vi "getPastFutureData.vi"(3 "2015 data future - R55 parsed.csv":path, 5 "2015 data past - R55 parsed.csv":path) -> (0 "Data Past Cluster":T1, 2 "Data Future Cluster":T2)   [LabVIEW 2013]
uses:
  <vilib>/Utility/file.llb/Read From Spreadsheet File (DBL).vi
panel:
  # "Daily Past Data       -7               -6              -5              -4              -3               -2              -1"
  # "Daily Future Data +1               +2              +3             +4             +5              +6              +7              +8             +9           +10            +11           +12"
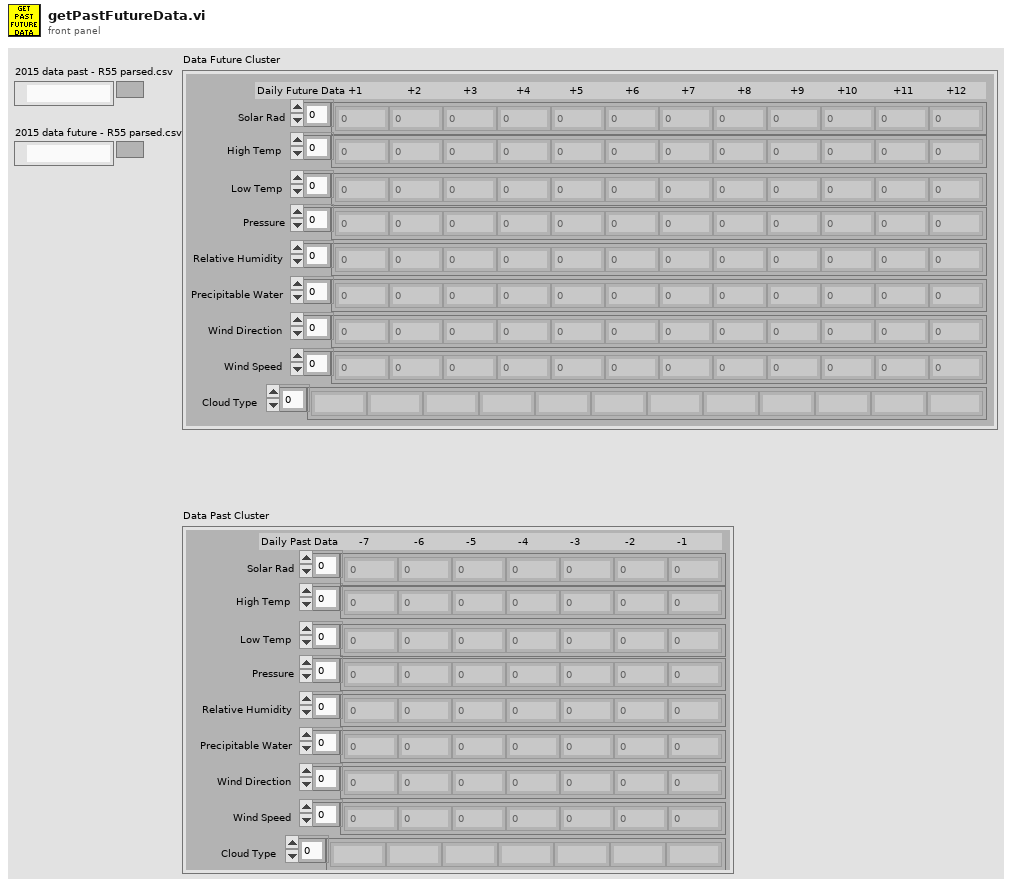
[diagram p1: front panel]
types:
  T1 = cluster{"Wind Speed":dbl[], "Wind Direction":dbl[], "Precipitable Water":dbl[], "Relative Humidity":dbl[], "Pressure":dbl[], "Low Temp":dbl[], "High Temp":dbl[], "Solar Rad":dbl[], "Cloud Type":string[]}
  T2 = cluster{"Solar Rad":dbl[], "High Temp":dbl[], "Low Temp":dbl[], "Pressure":dbl[], "Relative Humidity":dbl[], "Precipitable Water":dbl[], "Wind Direction":dbl[], "Wind Speed":dbl[], "Cloud Type":string[]}
  T3 = cluster{dbl[], dbl[], dbl[], dbl[], dbl[], dbl[], dbl[], dbl[], string[]}
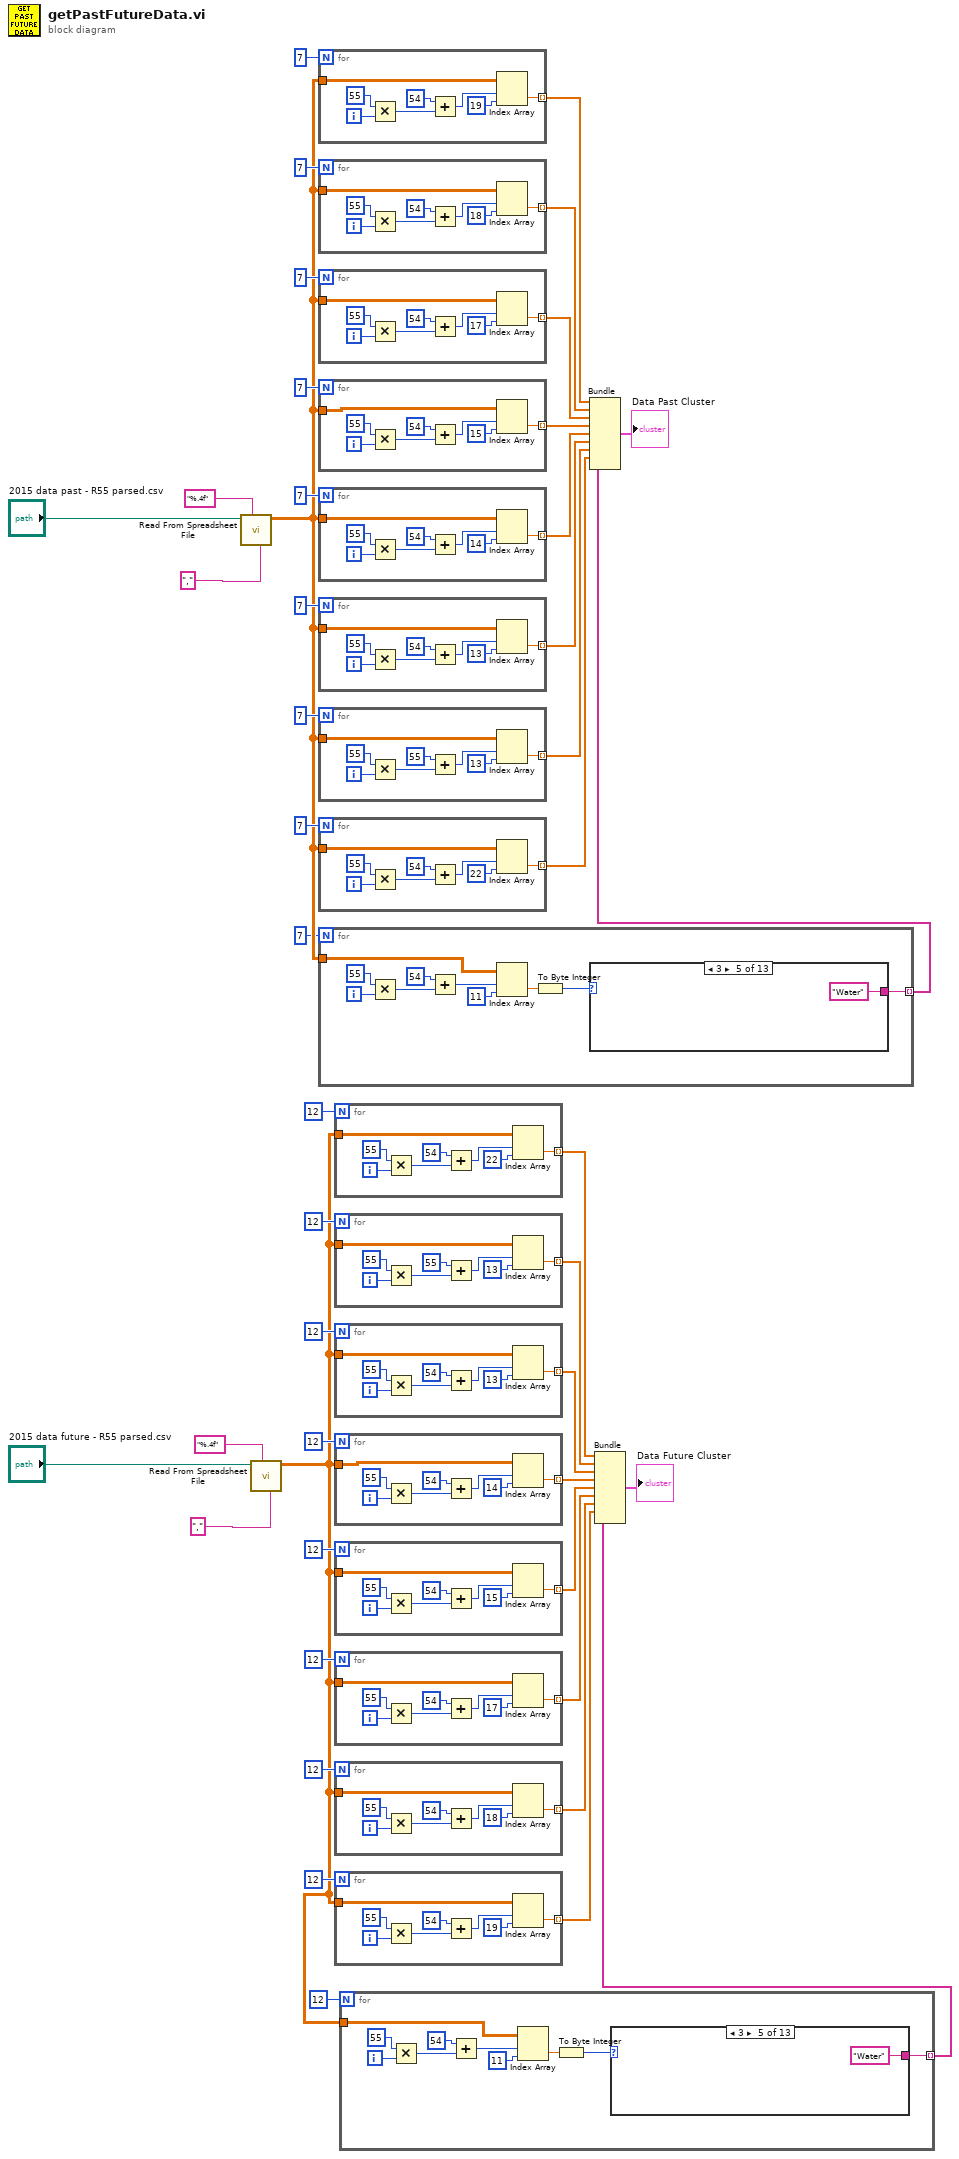
[diagram p0: block diagram]
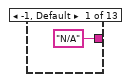
[diagram p2: hidden frame]
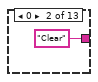
[diagram p3: hidden frame]
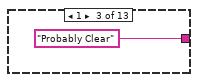
[diagram p4: hidden frame]
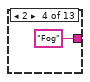
[diagram p5: hidden frame]
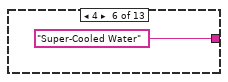
[diagram p6: hidden frame]
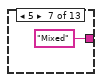
[diagram p7: hidden frame]
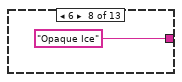
[diagram p8: hidden frame]
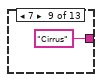
[diagram p9: hidden frame]
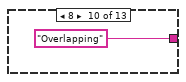
[diagram p10: hidden frame]
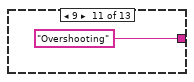
[diagram p11: hidden frame]
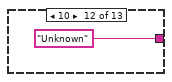
[diagram p12: hidden frame]
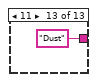
[diagram p13: hidden frame]
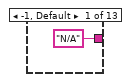
[diagram p14: hidden frame]
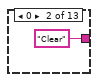
[diagram p15: hidden frame]
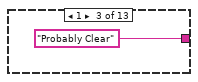
[diagram p16: hidden frame]
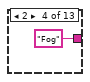
[diagram p17: hidden frame]
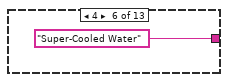
[diagram p18: hidden frame]
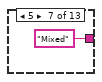
[diagram p19: hidden frame]
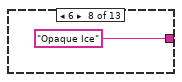
[diagram p20: hidden frame]
diagram:
  n1 = call-poly <vilib>:"Read From Spreadsheet File.vi"("delimiter (\\t)"="," ("delimiter (\\t)"), "format (%.3f)"="%.4f" ("format (%d)"), "file path (dialog if empty)"="2015 data past - R55 parsed.csv") -> ("all rows"=w6:dbl[][])  [unwired: 4 in, 4 out]
  n2 = call-poly <vilib>:"Read From Spreadsheet File.vi"("delimiter (\\t)"="," ("delimiter (\\t)"), "format (%.3f)"="%.4f" ("format (%d)"), "file path (dialog if empty)"="2015 data future - R55 parsed.csv") -> ("all rows"=w2:dbl[][])  [unwired: 4 in, 4 out]
  n3 = for {
    N: 7 -> [_]
    tunnel: w6 -> [w54]
    tunnel: [w47] -> w8 mode=indexing
    i -> [w51]
    n4 = Multiply(x=55, y=w51) -> (x*y=w52:i32)
    n5 = Add(x=54, y=w52) -> (x+y=w49:i32)
    n6 = Index Array(array=w54, index (row)=w49, index (col)=19 ("disabled index (col)")) -> (element=w47:dbl)
  }
  n7 = for {
    N: 7 -> [_]
    tunnel: w6 -> [w62]
    tunnel: [w55] -> w9 mode=indexing
    i -> [w59]
    n8 = Multiply(x=55, y=w59) -> (x*y=w60:i32)
    n9 = Add(x=54, y=w60) -> (x+y=w57:i32)
    n10 = Index Array(array=w62, index (row)=w57, index (col)=18 ("disabled index (col)")) -> (element=w55:dbl)
  }
  n11 = for {
    N: 7 -> [_]
    tunnel: w6 -> [w70]
    tunnel: [w63] -> w10 mode=indexing
    i -> [w67]
    n12 = Multiply(x=55, y=w67) -> (x*y=w68:i32)
    n13 = Add(x=54, y=w68) -> (x+y=w65:i32)
    n14 = Index Array(array=w70, index (row)=w65, index (col)=17 ("disabled index (col)")) -> (element=w63:dbl)
  }
  n15 = for {
    N: 7 -> [_]
    tunnel: w6 -> [w78]
    tunnel: [w71] -> w11 mode=indexing
    i -> [w75]
    n16 = Multiply(x=55, y=w75) -> (x*y=w76:i32)
    n17 = Add(x=54, y=w76) -> (x+y=w73:i32)
    n18 = Index Array(array=w78, index (row)=w73, index (col)=15 ("disabled index (col)")) -> (element=w71:dbl)
  }
  n19 = for {
    N: 7 -> [_]
    tunnel: w6 -> [w86]
    tunnel: [w79] -> w12 mode=indexing
    i -> [w83]
    n20 = Multiply(x=55, y=w83) -> (x*y=w84:i32)
    n21 = Add(x=54, y=w84) -> (x+y=w81:i32)
    n22 = Index Array(array=w86, index (row)=w81, index (col)=14 ("disabled index (col)")) -> (element=w79:dbl)
  }
  n23 = for {
    N: 7 -> [_]
    tunnel: w6 -> [w94]
    tunnel: [w87] -> w13 mode=indexing
    i -> [w91]
    n24 = Multiply(x=55, y=w91) -> (x*y=w92:i32)
    n25 = Add(x=54, y=w92) -> (x+y=w89:i32)
    n26 = Index Array(array=w94, index (row)=w89, index (col)=13 ("disabled index (col)")) -> (element=w87:dbl)
  }
  n27 = for {
    N: 7 -> [_]
    tunnel: w6 -> [w102]
    tunnel: [w95] -> w14 mode=indexing
    i -> [w99]
    n28 = Multiply(x=55, y=w99) -> (x*y=w100:i32)
    n29 = Add(x=55, y=w100) -> (x+y=w97:i32)
    n30 = Index Array(array=w102, index (row)=w97, index (col)=13 ("disabled index (col)")) -> (element=w95:dbl)
  }
  n31 = for {
    N: 7 -> [_]
    tunnel: w6 -> [w110]
    tunnel: [w103] -> w15 mode=indexing
    i -> [w107]
    n32 = Multiply(x=55, y=w107) -> (x*y=w108:i32)
    n33 = Add(x=54, y=w108) -> (x+y=w105:i32)
    n34 = Index Array(array=w110, index (row)=w105, index (col)=22 ("disabled index (col)")) -> (element=w103:dbl)
  }
  n35 = for {
    N: 7 -> [_]
    tunnel: w6 -> [w120]
    tunnel: [w111] -> w4 mode=indexing
    i -> [w117]
    n36 = Multiply(x=55, y=w117) -> (x*y=w118:i32)
    n37 = Add(x=54, y=w118) -> (x+y=w115:i32)
    n38 = Index Array(array=w120, index (row)=w115, index (col)=11 ("disabled index (col)")) -> (element=w112:dbl)
    n39 = To Byte Integer(number=w112) -> (8bit integer=w113:i8)
    n40 = case shown="3" w113 {
      tunnel: ["N/A" "Clear" "Probably Clear" "Fog" "Water" "Super-Cooled Water" "Mixed" "Opaque Ice" "Cirrus" "Overlapping" "Overshooting" "Unknown" "Dust"] -> w111
      frame -1, Default {
      }
      frame 0 {
      }
      frame 1 {
      }
      frame 2 {
      }
      frame 3 {
      }
      frame 4 {
      }
      frame 5 {
      }
      frame 6 {
      }
      frame 7 {
      }
      frame 8 {
      }
      frame 9 {
      }
      frame 10 {
      }
      frame 11 {
      }
    }
  }
  n41 = for {
    N: 12 -> [_]
    tunnel: w2 -> [w141]
    tunnel: [w134] -> w24 mode=indexing
    i -> [w138]
    n42 = Multiply(x=55, y=w138) -> (x*y=w139:i32)
    n43 = Add(x=54, y=w139) -> (x+y=w136:i32)
    n44 = Index Array(array=w141, index (row)=w136, index (col)=22 ("disabled index (col)")) -> (element=w134:dbl)
  }
  n45 = for {
    N: 12 -> [_]
    tunnel: w2 -> [w149]
    tunnel: [w142] -> w23 mode=indexing
    i -> [w146]
    n46 = Multiply(x=55, y=w146) -> (x*y=w147:i32)
    n47 = Add(x=55, y=w147) -> (x+y=w144:i32)
    n48 = Index Array(array=w149, index (row)=w144, index (col)=13 ("disabled index (col)")) -> (element=w142:dbl)
  }
  n49 = for {
    N: 12 -> [_]
    tunnel: w2 -> [w157]
    tunnel: [w150] -> w22 mode=indexing
    i -> [w154]
    n50 = Multiply(x=55, y=w154) -> (x*y=w155:i32)
    n51 = Add(x=54, y=w155) -> (x+y=w152:i32)
    n52 = Index Array(array=w157, index (row)=w152, index (col)=13 ("disabled index (col)")) -> (element=w150:dbl)
  }
  n53 = for {
    N: 12 -> [_]
    tunnel: w2 -> [w165]
    tunnel: [w158] -> w21 mode=indexing
    i -> [w162]
    n54 = Multiply(x=55, y=w162) -> (x*y=w163:i32)
    n55 = Add(x=54, y=w163) -> (x+y=w160:i32)
    n56 = Index Array(array=w165, index (row)=w160, index (col)=14 ("disabled index (col)")) -> (element=w158:dbl)
  }
  n57 = for {
    N: 12 -> [_]
    tunnel: w2 -> [w173]
    tunnel: [w166] -> w20 mode=indexing
    i -> [w170]
    n58 = Multiply(x=55, y=w170) -> (x*y=w171:i32)
    n59 = Add(x=54, y=w171) -> (x+y=w168:i32)
    n60 = Index Array(array=w173, index (row)=w168, index (col)=15 ("disabled index (col)")) -> (element=w166:dbl)
  }
  n61 = for {
    N: 12 -> [_]
    tunnel: w2 -> [w181]
    tunnel: [w174] -> w19 mode=indexing
    i -> [w178]
    n62 = Multiply(x=55, y=w178) -> (x*y=w179:i32)
    n63 = Add(x=54, y=w179) -> (x+y=w176:i32)
    n64 = Index Array(array=w181, index (row)=w176, index (col)=17 ("disabled index (col)")) -> (element=w174:dbl)
  }
  n65 = for {
    N: 12 -> [_]
    tunnel: w2 -> [w189]
    tunnel: [w182] -> w18 mode=indexing
    i -> [w186]
    n66 = Multiply(x=55, y=w186) -> (x*y=w187:i32)
    n67 = Add(x=54, y=w187) -> (x+y=w184:i32)
    n68 = Index Array(array=w189, index (row)=w184, index (col)=18 ("disabled index (col)")) -> (element=w182:dbl)
  }
  n69 = for {
    N: 12 -> [_]
    tunnel: w2 -> [w197]
    tunnel: [w190] -> w17 mode=indexing
    i -> [w194]
    n70 = Multiply(x=55, y=w194) -> (x*y=w195:i32)
    n71 = Add(x=54, y=w195) -> (x+y=w192:i32)
    n72 = Index Array(array=w197, index (row)=w192, index (col)=19 ("disabled index (col)")) -> (element=w190:dbl)
  }
  n73 = for {
    N: 12 -> [_]
    tunnel: w2 -> [w207]
    tunnel: [w198] -> w1 mode=indexing
    i -> [w204]
    n74 = Multiply(x=55, y=w204) -> (x*y=w205:i32)
    n75 = Add(x=54, y=w205) -> (x+y=w202:i32)
    n76 = Index Array(array=w207, index (row)=w202, index (col)=11 ("disabled index (col)")) -> (element=w199:dbl)
    n77 = To Byte Integer(number=w199) -> (8bit integer=w200:i8)
    n78 = case shown="3" w200 {
      tunnel: ["N/A" "Clear" "Probably Clear" "Fog" "Water" "Super-Cooled Water" "Mixed" "Opaque Ice" "Cirrus" "Overlapping" "Overshooting" "Unknown" "Dust"] -> w198
      frame -1, Default {
      }
      frame 0 {
      }
      frame 1 {
      }
      frame 2 {
      }
      frame 3 {
      }
      frame 4 {
      }
      frame 5 {
      }
      frame 6 {
      }
      frame 7 {
      }
      frame 8 {
      }
      frame 9 {
      }
      frame 10 {
      }
      frame 11 {
      }
    }
  }
  n79 = Bundle(w8, w9, w10, w11, w12, w13, w14, w15, w4) -> (→"Data Past Cluster":T3)  [unwired: 1 in]
  n80 = Bundle(w24, w23, w22, w21, w20, w19, w18, w17, w1) -> (→"Data Future Cluster":T3)  [unwired: 1 in]
